vi "ROI grp-Save to text file.vi"(11 "Groups setup to add/update":T1[](array[typedef]) {"Group region specifier cluster"."Contours"."Type" items=["No Selection", "Point", "Line", "Rectangle", "Oval", "Polygon", "Freehand Region", "Annulus", "Unused2", "Unused3", "Broken Line", "Freehand Line", "Rotated Rectangle"]}) -> (0 "error out":errorcluster)   [LabVIEW 2017]
uses:
  ROI Selection Interface/ROI group info cluster.ctl
  Experiment header interface/Typedefs/Save-Load-Save as-Load last enum.ctl
panel:
  out "Array":string[][](array[string])
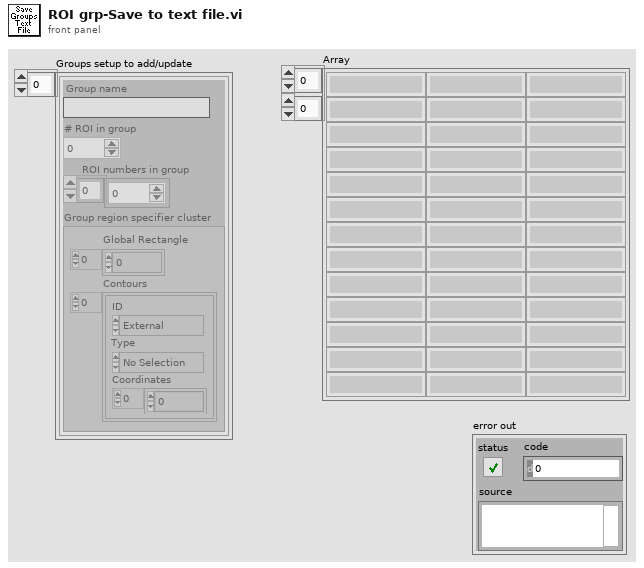
[diagram p1: front panel]
types:
  T1 = typedef "ROI group info cluster.ctl" = cluster{"Group name":string, "# ROI in group":i32, "ROI numbers in group":i32[], "Group region specifier cluster":T2}
  T2 = typedef "ROI Descriptor" = cluster{"Global Rectangle":i32[], "Contours":cluster{"ID":enum32{"External", "Internal"}, "Type":u32, "Coordinates":i32[]}[]}
  T3 = typedef "Save-Load-Save as-Load last enum.ctl" = enum16{"Save file", "Save file as", "Load file", "Load last file"}
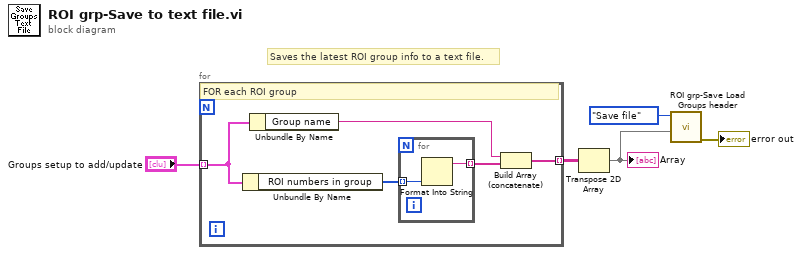
[diagram p0: block diagram]
diagram:
  # "Saves the latest ROI group info to a text file."
  n1 = for {
    tunnel: "Groups setup to add/update" -> [w10] mode=indexing
    tunnel: [w6] -> w4 mode=indexing
    # "FOR each ROI group"
    n2 = Unbundle By Name(w10) -> ("ROI numbers in group"=w9:i32[])
    n3 = Unbundle By Name(w10) -> ("Group name"=w7:string)
    n4 = for {
      tunnel: w9 -> [w12] mode=indexing
      tunnel: [w11] -> w8 mode=indexing
      n5 = Format Into String(w12) -> (resulting string=w11:string)  [unwired: 3 in, 1 out]
    }
    n6 = Build Array (concatenate)(w7, w8) -> (w6:string[])
  }
  n7 = Transpose 2D Array(2D array=w4) -> (transposed array=w3:string[][])
  "Array" <- w3
  n8 = call "ROI grp-Save Load Groups header.vi"("POI groups header file data (in)"=w3, "Function"=Save-Load-Save_as-Load_last_enum."Save file") -> ("error out"=→"error out":errorcluster)  [unwired: 7 in, 2 out]
